vi "PWM51.vi"() -> ()   [LabVIEW 2019]
uses:
  <vilib>/rvi/Emulation/niFpgaGetClockAttributes.vi
  <vilib>/rvi/Emulation/niFpgaSctlEmulationGetInTimedLoop.vi
  <vilib>/rvi/Emulation/niFpgaEmulationReportErrorSimple.vi
  <vilib>/rvi/eio/common/nirviEmuTemplateMethod_errors.vi
  <vilib>/rvi/Emulation/niFpgaCriticalErrorInLSC.vi
  <vilib>/eio/EIONode/EIONode.xnode
panel:
  out "x-1":sgl format="%#_7g"
  out "波形图表":sgl(graph)
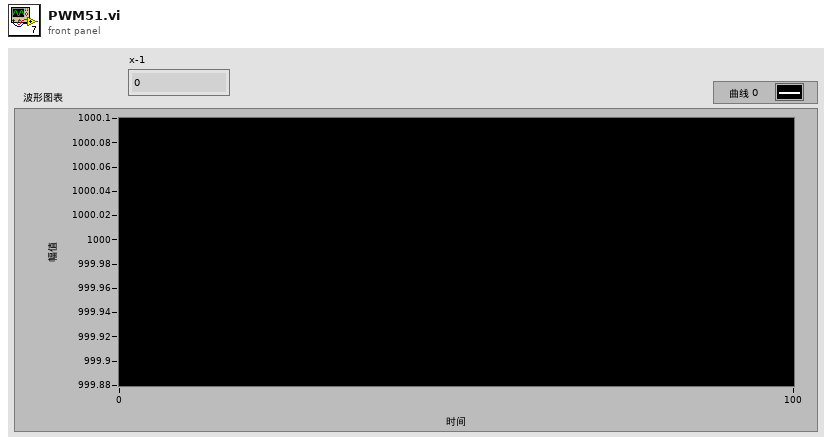
[diagram p1: front panel]
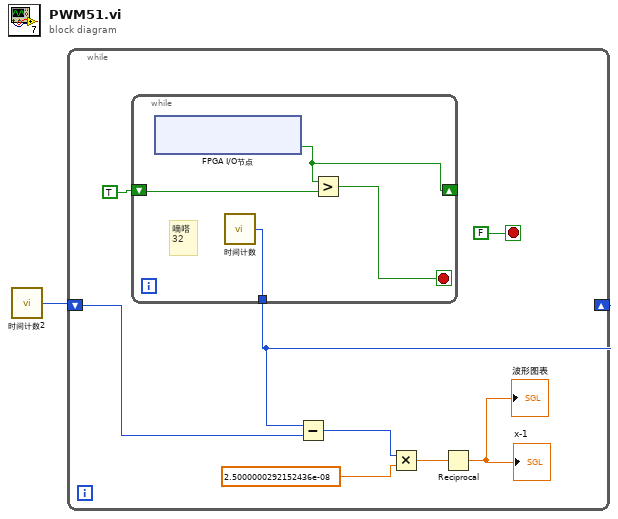
[diagram p0: block diagram]
diagram:
  n1 = call "时间计数2"() -> ("Tick Count(Ticks)"=w1:u32)
  n2 = while {
    shift-right: [w7] -> _
    shift-left: w1 -> [w6]
    stop <- FALSE stop-if-true
    n3 = while {
      shift-right: [w12] -> _
      shift-left: TRUE -> [w13]
      tunnel: [w10] -> w7
      stop <- w11 stop-if-true
      # "嘀嗒\n32"
      n4 = xnode "FPGA I/O节点"() -> ("ConnectorB/DIO0"=w12:bool)  [unwired: 1 in, 1 out]
      n5 = call "时间计数"() -> ("Tick Count(Ticks)"=w10:u32)
      n6 = Greater?(x=w12, y=w13) -> (0:w11:bool)
    }
    n7 = Subtract(x=w7, y=w6) -> (x-y=w5:u32)
    n8 = Multiply(x=w5, y=sgl 2.5e-08) -> (x*y=w3:sgl)
    n9 = Reciprocal(x=w3) -> (1/x=→"x-1" →"波形图表":sgl)
  }
